vi "Find Common Path.vi"(8 "error in (no error)":errorcluster, 11 "File Paths":path[](array[path])) -> (0 "error out":errorcluster, 3 "Common Path":path)   [LabVIEW 2020, in "File Tree.lvclass"]
uses:
  File Tree.lvclass
  File Tree.lvclass/File Tree.ctl
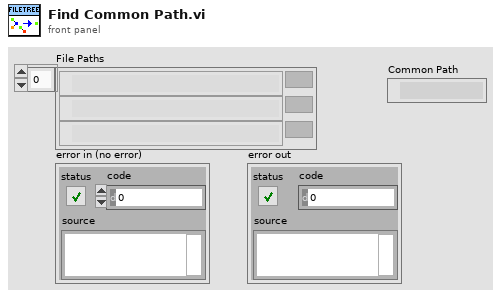
[diagram p1: front panel]
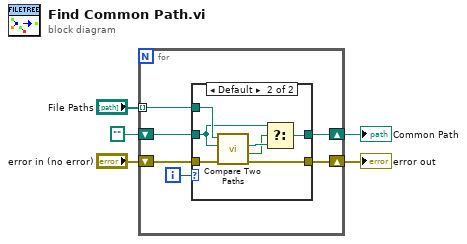
[diagram p0: block diagram]
diagram:
  n1 = for {
    tunnel: "File Paths" -> [w11] mode=indexing
    shift-right: [w8] -> w1
    shift-left: path "" ("Empty Path Constant") -> [w7]
    shift-right: [w10] -> w4
    shift-left: "error in (no error)" -> [w9]
    i -> [w6]
    n2 = case shown="Default" w6 {
      tunnel: w11 -> [w12 w20]
      tunnel: [w13 w19] -> w10
      tunnel: w9 -> [w13 w18]
      tunnel: [w12 w14] -> w8
      tunnel: w7 -> [_ w15]
      frame 0 {
      }
      frame Default {
        n3 = call <vilib>:"Compare Two Paths.vi"("error in (no error)"=w18, "Path 2"=w15, "Path 1"=w20) -> ("error out"=w19:errorcluster, "Path 2 Relative to Path 1?"=w16:bool, "Common Path"=w17:path)  [unwired: 5 in, 1 out]
        n4 = Select(t=w15, s=w16, f=w17) -> (s? t:f=w14:path)
      }
    }
  }
  "error out" <- w4
  "Common Path" <- w1
